vi "FiringCylinder7.vi"(7 "Action":T4, 8 "error in (no error)":errorcluster, 9 "Default Position":bool, 10 "Actuate?":bool, 11 "SolenoidDevRef":T1={"DevStatus"={"status"=FALSE, "code"=0, "source"=""}, "Solenoid Module"=enum."Solenoid Module 1", "Forward Solenoid Channel"=enum."Invalid", "Reverse Solenoid Channel"=enum."Invalid"}) -> (0 "error out":errorcluster)   [LabVIEW 2013]
doc: "Controls a single solenoid. It has the following actions:\n-Init: takes a reference to a single solenoid and stores it in a shift register so that the reference does not need to be passed again. Also takes a boolean for default position: if default position is false (the \"normal\" case), then Off corresponds to the retracted state and On corresponds to the actuated state. If default position is true, then Off corresponds to the *actuated* state and On corresponds to the *retracted* state.\n-SetValue: sets the position of the solenoid. True actuates the solenoid, false retracts it.\n-Disable: sets the solenoid to the retracted position."
uses:
  Robot_Framework_2014/SingleSolenoidAction.ctl
  <vilib>/Rock Robotics/WPI/Solenoid/WPI_SolenoidDevRef.ctl
  <vilib>/Rock Robotics/SystemInterfaces/Typedef/FPGA_TypedefSolenoidModule.ctl
  <vilib>/Rock Robotics/WPI/Solenoid/WPI_SolenoidChannel.ctl
  <vilib>/Rock Robotics/WPI/Solenoid/WPI_SolenoidValue.ctl
  <vilib>/Rock Robotics/WPI/Solenoid/WPI_SolenoidSetEnum.vi
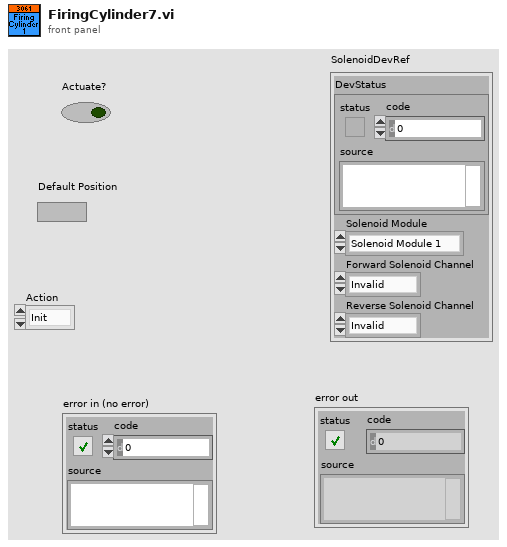
[diagram p1: front panel]
types:
  T1 = typedef "WPI_SolenoidDevRef.ctl" = cluster{"DevStatus":errorcluster, "Solenoid Module":T2, "Forward Solenoid Channel":T3, "Reverse Solenoid Channel":T3}
  T2 = typedef "FPGA_TypedefSolenoidModule.ctl" = enum16{"Solenoid Module 1", "Solenoid Module 2"}
  T3 = typedef "WPI_SolenoidChannel.ctl" = enum8{"Solenoid 1", "Solenoid 2", "Solenoid 3", "Solenoid 4", "Solenoid 5", "Solenoid 6", "Solenoid 7", "Solenoid 8", "Invalid"}
  T4 = typedef "SingleSolenoidAction.ctl" = enum16{"Init", "SetState", "Disable"}
  T5 = typedef "WPI_SolenoidValue.ctl" = enum16{"Off", "On", "Forward", "Reverse"}
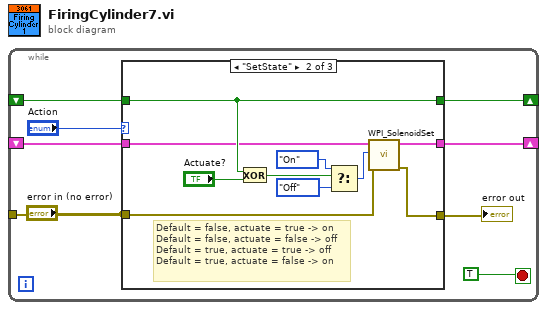
[diagram p0: block diagram]
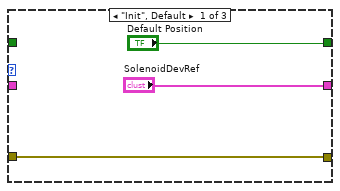
[diagram p2: hidden frame]
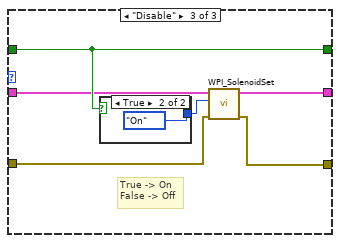
[diagram p3: hidden frame]
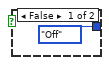
[diagram p4: hidden frame]
diagram:
  n1 = while {
    shift-right: [w6] -> _
    shift-left: _ -> [w8]
    shift-right: [w4] -> _
    shift-left: _ -> [w3]
    tunnel: ["error in (no error)"] -> _
    stop <- TRUE stop-if-true
    n2 = case shown="\"SetState\"" "Action" {
      tunnel: w8 -> [_ w20 w26]
      tunnel: ["Default Position" w20 w26] -> w6
      tunnel: ["SolenoidDevRef" w18 w24] -> w4
      tunnel: w3 -> [_ w19 w25]
      tunnel: "error in (no error)" -> [w11 w17 w23]
      tunnel: [w11 w16 w22] -> w1
      frame "Init", Default {
      }
      frame "SetState" {
        # "Default = false, actuate = true -> on\nDefault = false, actuate = false -> off\nDefault = true, actuate = true -> off\nDefault = true, actuate = false -> on"
        n3 = Exclusive Or(1:"Actuate?", 2:w20) -> (0:w13:bool)
        n4 = Select(t=WPI_SolenoidValue."On" ("Value"), s=w13, f=WPI_SolenoidValue."Off" ("Value")) -> (s? t:f=w12:T5)
        n5 = call-poly <vilib>:"WPI_SolenoidSet.vi"("error in (no error)"=w17, "Value"=w12, "SolenoidDevRef"=w19) -> ("error out"=w16:errorcluster, "SolenoidDevRef"=w18:T1)  [unwired: 7 in]
      }
      frame "Disable" {
        # "True -> On\nFalse -> Off"
        n6 = case shown="True" w26 {
          tunnel: [WPI_SolenoidValue."Off" ("Value") WPI_SolenoidValue."On" ("Value")] -> w27
          frame False {
          }
          frame True {
          }
        }
        n7 = call-poly <vilib>:"WPI_SolenoidSet.vi"("error in (no error)"=w23, "Value"=w27, "SolenoidDevRef"=w25) -> ("error out"=w22:errorcluster, "SolenoidDevRef"=w24:T1)  [unwired: 7 in]
      }
    }
    "error out" <- w1
  }
